vi "New_Magazine_Set.vi"   [LabVIEW 2019]
uses:
  New_Magazine_Control_States.ctl
  New_Magazine_Globals.vi
  Flywheel/Flywheel_Globals.vi
types:
  T1 = typedef "New_Magazine_Control_States.ctl" = enum16{"No-Op", "Up", "Down", "Manual", "Fire", "Spinning Up"}
  T2 = typedef "New_Magazine_Cluster.ctl" = cluster{"Control_States":T1, "Firing":bool, "Throttle":dbl, "Spinning Up":bool, "Off":bool}
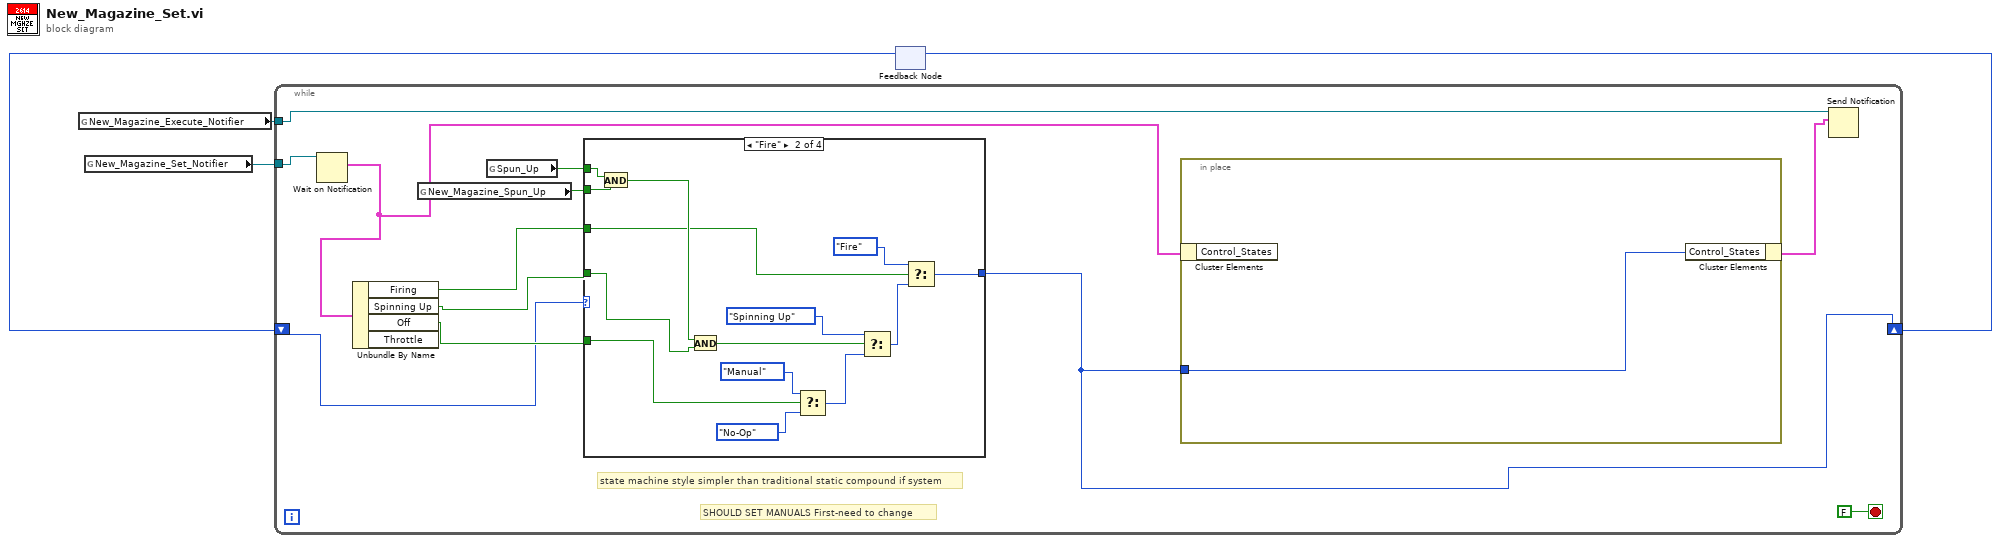
[diagram p0: block diagram]
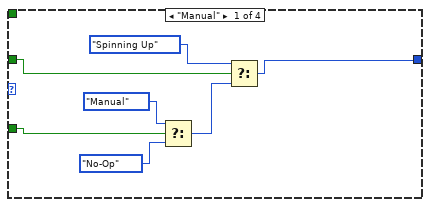
[diagram p2: hidden frame]
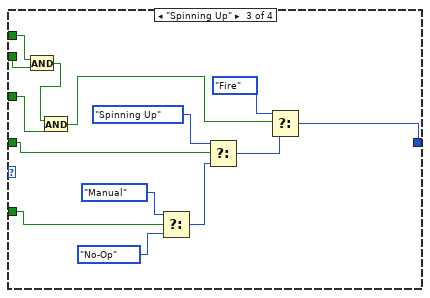
[diagram p3: hidden frame]
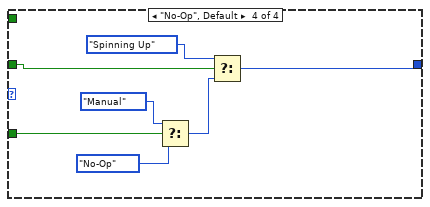
[diagram p4: hidden frame]
diagram:
  n1 = global read "New_Magazine_Globals.vi" "New_Magazine_Execute_Notifier"() -> (w4:refnum<notifier>)
  n2 = global read "New_Magazine_Globals.vi" "New_Magazine_Set_Notifier"() -> (w1:refnum<notifier>)
  n3 = feedback #1() -> (w2:T1)  [unwired: 1 in]
  n4 = while {
    tunnel: w4 -> [w15]
    shift-right: [w7] -> w3
    shift-left: w2 -> [w8]
    tunnel: w1 -> [w14]
    stop <- FALSE stop-if-true
    # "SHOULD SET MANUALS First-need to change"
    # "state machine style simpler than traditional static compound if system"
    n5 = Wait on Notification(notifier=w14) -> (notification=w13:T2)  [unwired: 3 in, 3 out]
    n6 = Unbundle By Name(w13) -> ("Firing"=w9:bool, "Spinning Up"=w10:bool, "Off"=w11:bool)  [unwired: 1 out]
    n7 = global read "New_Magazine_Globals.vi" "New_Magazine_Spun_Up"() -> (w5:bool)
    n8 = global read "Flywheel_Globals.vi" "Spun_Up"() -> (w6:bool)
    n9 = case shown="\"Fire\"" w8 {
      tunnel: w11 -> [w18 w30 w47 w53]
      tunnel: w10 -> [w17 w27 w41 w52]
      tunnel: w9 -> [_ w25 w38 _]
      tunnel: [w19 w31 w39 w54] -> w7
      tunnel: w6 -> [_ w29 w46 _]
      tunnel: w5 -> [_ w24 w44 _]
      frame "Manual" {
        n10 = Select(t=New_Magazine_Control_States."Manual" ("Control_States"), s=w18, f=New_Magazine_Control_States."No-Op" ("Control_States")) -> (s? t:f=w23:T1)
        n11 = Select(t=New_Magazine_Control_States."Spinning Up" ("Control_States"), s=w17, f=w23) -> (s? t:f=w19:T1)
      }
      frame "Fire" {
        n12 = And(x=w29, y=w24) -> (x .and. y?=w28:bool)
        n13 = And(x=w28, y=w27) -> (x .and. y?=w26:bool)
        n14 = Select(t=New_Magazine_Control_States."Manual" ("Control_States"), s=w30, f=New_Magazine_Control_States."No-Op" ("Control_States")) -> (s? t:f=w37:T1)
        n15 = Select(t=New_Magazine_Control_States."Spinning Up" ("Control_States"), s=w26, f=w37) -> (s? t:f=w33:T1)
        n16 = Select(t=New_Magazine_Control_States."Fire" ("Control_States"), s=w25, f=w33) -> (s? t:f=w31:T1)
      }
      frame "Spinning Up" {
        n17 = And(x=w46, y=w44) -> (x .and. y?=w45:bool)
        n18 = And(x=w45, y=w38) -> (x .and. y?=w40:bool)
        n19 = Select(t=New_Magazine_Control_States."Manual" ("Control_States"), s=w47, f=New_Magazine_Control_States."No-Op" ("Control_States")) -> (s? t:f=w49:T1)
        n20 = Select(t=New_Magazine_Control_States."Spinning Up" ("Control_States"), s=w41, f=w49) -> (s? t:f=w43:T1)
        n21 = Select(t=New_Magazine_Control_States."Fire", s=w40, f=w43) -> (s? t:f=w39:T1)
      }
      frame "No-Op", Default {
        n22 = Select(t=New_Magazine_Control_States."Manual" ("Control_States"), s=w53, f=New_Magazine_Control_States."No-Op" ("Control_States")) -> (s? t:f=w56:T1)
        n23 = Select(t=New_Magazine_Control_States."Spinning Up" ("Control_States"), s=w52, f=w56) -> (s? t:f=w54:T1)
      }
    }
    n24 = in-place {
      in-place-border: w7 -> [w59]
      n25 = in-place-cluster #2(w13) -> ()  [unwired: 1 out]
      n26 = in-place-cluster #2("Control_States"=w59) -> (w12:T2)
    }
    n27 = Send Notification(notification=w12, notifier=w15) -> ()  [unwired: 1 in, 2 out]
  }
  n28 = feedback-in #1(w3) -> ()
